vi "Align Buffers.vi"(8 "error in (no error)":errorcluster, 10 "base Inline Buffer":refnum<class "Buffer.lvclass">, 11 "Transfer Group in":refnum<class "Transfer Group.lvclass">) -> (0 "error out":errorcluster, 3 "Transfer Group out":refnum<class "Transfer Group.lvclass">)   [LabVIEW 2019, in "DSF Core.lvlib" / "Transfer Group.lvclass"]
uses:
  Transfer Group.lvclass
  Buffer/Buffer.lvclass
  C:/Program Files (x86)/National Instruments/LabVIEW 2019/vi.lib/NI/Memory Manager/Classes/Pointer/Pointer.lvclass
  Transfer Group.lvclass/Transfer Group.ctl
  Buffers/Buffers.lvclass/Buffers.ctl
  <vilib>/NI/Memory Manager/Classes/Pointer/Pointer.lvclass/Pointer.ctl
  Buffer/Buffer.lvclass/Buffer.ctl
  Transfer/Transfer.lvclass/Transfer.ctl
  Buffer/Align to Base Buffer.vi
  <vilib>/NI/Memory Manager/Classes/Pointer/Get Address.vi
  <vilib>/NI/Memory Manager/Classes/Pointer/Encapsulate.vi
  <vilib>/NI/Memory Manager/Classes/Pointer/Get Size.vi
  <vilib>/NI/Memory Manager/Classes/Pointer/Is Null.vi
  <vilib>/NI/Memory Manager/Classes/Pointer/Set Size.vi
  <vilib>/NI/Memory Manager/Classes/Pointer/Set Address.vi
  <vilib>/NI/Memory Manager/Classes/Pointer/Check Null Pointer.vi
  <vilib>/NI/Memory Manager/Classes/Pointer/Set Internal.vi
  <vilib>/NI/Memory Manager/Classes/Pointer/Errors.vi
  <vilib>/NI/Memory Manager/Classes/Pointer/Null Pointer.vi
  <vilib>/NI/Memory Manager/Classes/Pointer/Create Error.vi
  <vilib>/NI/Memory Manager/VIs/New Error Cluster.vi
  <vilib>/NI/Memory Manager/VIs/New Error Cluster (512B).vi
  <vilib>/NI/Memory Manager/VIs/Set Error Status.vi
  <vilib>/NI/Memory Manager/VIs/Set Error Code.vi
  <vilib>/NI/Memory Manager/VIs/Set Error Source.vi
  <vilib>/NI/Memory Manager/Constants/Constants.vi
  <vilib>/NI/Memory Manager/Constants/Library Name.vi
  <vilib>/NI/Memory Manager/Classes/Pointer/Pointer Error Info.vi
  <vilib>/NI/Memory Manager/VIs/Write String to Source.vi
  <vilib>/NI/Memory Manager/Constants/Pointer Class Name.vi
  Transfer/Transfer.lvclass
  Buffers/Buffers.lvclass
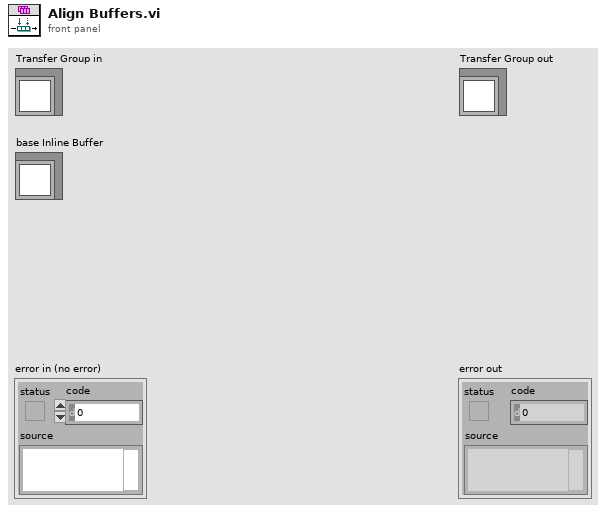
[diagram p1: front panel]
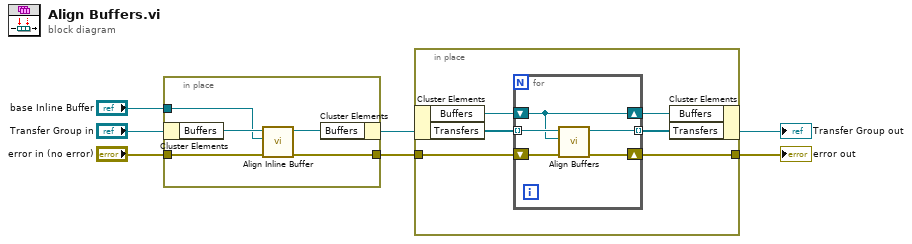
[diagram p0: block diagram]
diagram:
  n1 = in-place {
    in-place-border: "error in (no error)" -> [w12]
    in-place-border: [w11] -> w1
    in-place-border: "base Inline Buffer" -> [w8]
    n2 = in-place-cluster #1("Transfer Group in") -> ("Buffers"=w10:refnum<class "Buffers.lvclass">)
    n3 = call "Align Inline Buffer.vi"("error in (no error)"=w12, "base Inline Buffer"=w8, "Buffers in"=w10) -> ("error out"=w11:errorcluster, "Buffers out"=w9:refnum<class "Buffers.lvclass">)  [unwired: 7 in]
    n4 = in-place-cluster #1("Buffers"=w9) -> (w3:refnum<class "Transfer Group.lvclass">)
  }
  n5 = in-place {
    in-place-border: [w16] -> w7
    in-place-border: w1 -> [w15]
    n6 = in-place-cluster #2(w3) -> ("Buffers"=w14:refnum<class "Buffers.lvclass">, "Transfers"=w18:refnum<class "Transfer.lvclass">[])
    n7 = for {
      tunnel: w18 -> [w23] mode=indexing
      tunnel: [w21] -> w17 mode=indexing
      shift-right: [w20] -> w16
      shift-left: w15 -> [w22]
      shift-right: [w19] -> w13
      shift-left: w14 -> [w19]
      n8 = call "Align Buffers.vi"("error in (no error)"=w22, "Transfer Group Buffers"=w19, "Transfer in"=w23) -> ("error out"=w20:errorcluster, "Transfer out"=w21:refnum<class "Transfer.lvclass">)  [unwired: 7 in]
    }
    n9 = in-place-cluster #2("Buffers"=w13, "Transfers"=w17) -> (→"Transfer Group out":refnum<class "Transfer Group.lvclass">)
  }
  "error out" <- w7
